vi "Write BG_level.vi"(8 "error in (no error)":errorcluster, 10 "BG_level":i32=-1, 11 "VIS-IR in":refnum<class "VIS-IR.lvclass">) -> (0 "error out":errorcluster, 3 "VIS-IR out":refnum<class "VIS-IR.lvclass">)   [LabVIEW 2015, in "VIS-IR.lvclass"]
uses:
  VIS-IR.lvclass
  Detector.lvclass
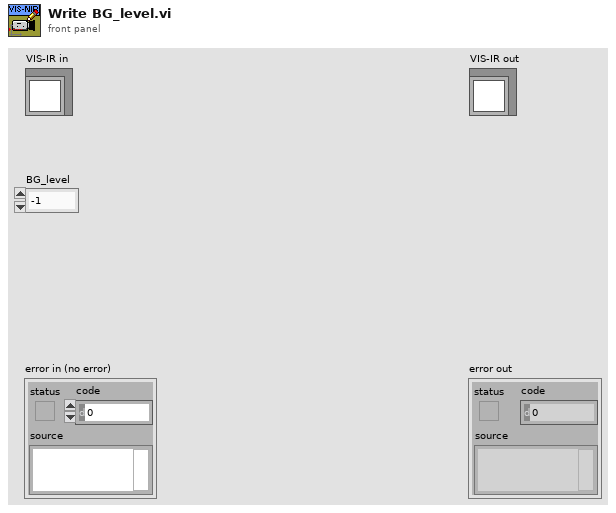
[diagram p1: front panel]
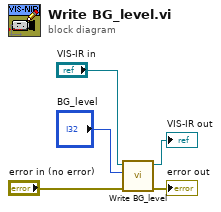
[diagram p0: block diagram]
diagram:
  n1 = call-parent "Write BG_level.vi"("error in (no error)"="error in (no error)", "BG_level"="BG_level", "Detector in"="VIS-IR in") -> ("error out"=→"error out":errorcluster, "Detector out"=→"VIS-IR out":refnum<class "VIS-IR.lvclass">)  [unwired: 7 in]
